vi "SHAPE_GA_Calculate Fitnesses.vi"(6 "Parameters":T1={"Population size"=100, "Generations no."=500, "Significant digits"=4, "Crossover probabality"=0.85, "Mutation mode"=enum."one-point, fixed rate", "Use Gray code?"=FALSE, "Mutation rate"=0.05, "Min mutation rate"=0.0005, "Max mutation rate"=0.25, "Reproduction plan"=enum."Steady-state-replace-worst", "Elitism"=FALSE, "Fmax"=1} {"Max mutation rate" min=0.0 max=1.0; "Min mutation rate" min=0.0 max=1.0; "Mutation rate" min=0.0 max=1.0; "Crossover probabality" min=0.0 max=1.0; "Significant digits" min=1; "Generations no." min=1; "Population size" min=1}, 7 "Fitness Function":T3, 11 "Population in":T2) -> (3 "Population out":T2)   [LabVIEW 2016, in "Shapelets Search (GA).lvlib"]
doc: "Рассчитать значения функции приспособленности"
uses:
  Shapelets Search (GA).lvlib
  5. Features Optimization/_Optimal Frequency Bands Search/GA_core/GA_tFitness Function.ctl
  5. Features Optimization/_Optimal Frequency Bands Search/GA_core/GA_tPopulation.ctl
  5. Features Optimization/_Optimal Frequency Bands Search/GA_core/GA_tParameters.ctl
  5. Features Optimization/_Optimal Frequency Bands Search/GA_core/GeneticAlgorithm.lvlib
panel:
  # "This VI is a part of BCI Design library, http://www.ru-bci.org \nCopyright © 2020, Sotnikov Peter, All rights reserved. License: GNU GPLv3"
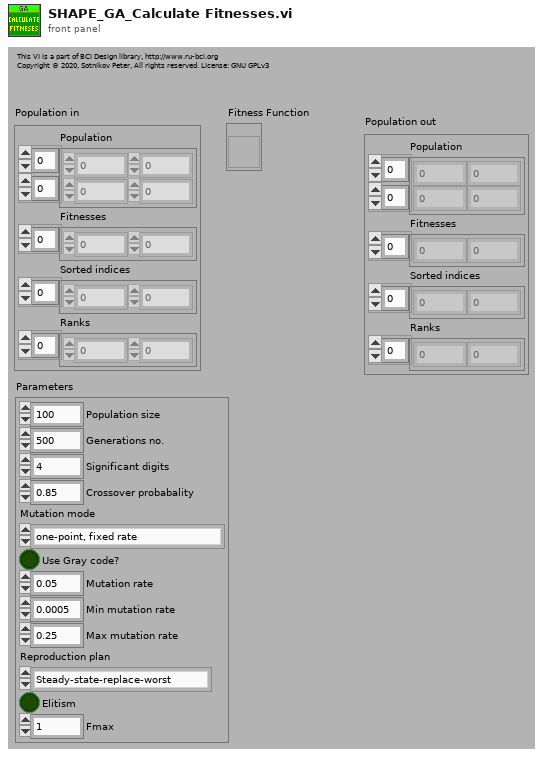
[diagram p1: front panel]
types:
  T1 = typedef "Optimal Frequency Bands Search.lvlib/GeneticAlgorithm.lvlib/GA_tParameters.ctl" = cluster{"Population size":i32, "Generations no.":i32, "Significant digits":i32, "Crossover probabality":dbl, "Mutation mode":enum16{"one-point, fixed rate", "one-point, fitness-adjustable rate", "one-point, distance-adjustable rate"}, "Use Gray code?":bool, "Mutation rate":dbl, "Min mutation rate":dbl, "Max mutation rate":dbl, "Reproduction plan":enum16{"Full generational replacement", "Steady-state-replace-random", "Steady-state-replace-worst"}, "Elitism":bool, "Fmax":i32}
  T2 = typedef "Optimal Frequency Bands Search.lvlib/GeneticAlgorithm.lvlib/GA_tPopulation.ctl" = cluster{"Population":i32[][], "Fitnesses":dbl[], "Sorted indices":i32[], "Ranks":i32[]}
  T3 = typedef "Optimal Frequency Bands Search.lvlib/GeneticAlgorithm.lvlib/GA_tFitness Function.ctl" = refnum<vi>
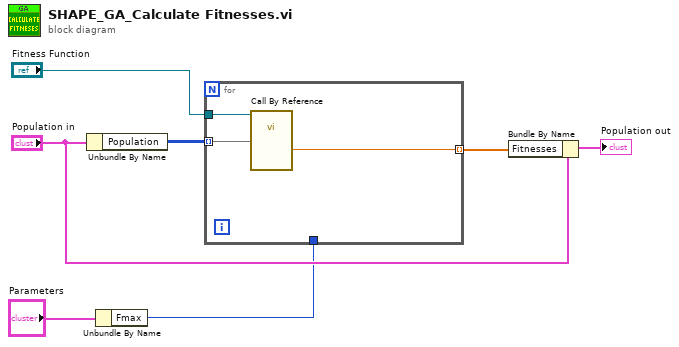
[diagram p0: block diagram]
diagram:
  n1 = Unbundle By Name("Population in") -> ("Population"=w7:i32[][])
  n2 = Unbundle By Name("Parameters") -> ("Fmax"=w2:i32)
  n3 = for {
    tunnel: w7 -> [w9] mode=indexing
    tunnel: "Fitness Function" -> [w10]
    tunnel: w2 -> [_]
    tunnel: [w8] -> w1 mode=indexing
    n4 = call-by-ref "Call By Reference"(reference=w10, "Phenotype"=w9) -> ("Fitness"=w8:dbl)  [unwired: 3 in, 2 out]
  }
  n5 = Bundle By Name(cluster="Population in", "Fitnesses"=w1) -> (→"Population out":T2)
